vi "Drop Parameters.vi"(6 "Main UI Message Queue":refnum<queue>, 7 "Mouse Position":cluster{"X":i32, "Y":i32}, 8 "error in (no error)":errorcluster, 9 "Parent Window Title":string, 10 "Module Type":T1=enum."Feed", 11 "State in":T2 {"Main Config"."PR Module Configs"."Settings"."PID 2 Parameters"."output range"."output low" format="%.2f"; "Main Config"."PR Module Configs"."Settings"."PID 2 Parameters"."output range"."output high" min=0.0 max=100.0 format="%.2f"; "Main Config"."PR Module Configs"."Settings"."PID 2 Parameters"."PID gains"."derivative time (Td, min)" format="%.3f"; "Main Config"."PR Module Configs"."Settings"."PID 2 Parameters"."PID gains"."integral time (Ti, min)" format="%.3f"; "Main Config"."PR Module Configs"."Settings"."PID 2 Parameters"."PID gains"."proportional gain (Kc)" format="%.3f"; "Main Config"."Steps"."Control" items=["Pump %", "Setpoint"]; "Main Config"."TCU Module Configs"."Settings"."Huber Unistat 410 Settings"."Address" min=0 max=99 format="%02.0f"; "Main Config"."TCU Module Configs"."Settings"."Julabo FP-50 Settings"."Pump Power" min=0 max=8 step=1; "Main Config"."TCU Module Configs"."Settings"."Lauda Settings"."Pump Power" min=0 max=8 step=1; "Main Config"."Pump Module Configs"."Settings"."ASIA Pump C"."channel" min=0 max=1 step=1; "Main Config"."Pump Module Configs"."Settings"."Masterflex"."Pump Number" min=1.0 max=20.0 step=1.0; "Main Config"."Pump Module Configs"."Settings"."Ismatech"."Pump Number" min=1.0 max=20.0 step=1.0; "Main Config"."Feed Module Configs"."Settings"."output range"."output low" min=0.0 max=100.0 format="%.2f"; "Main Config"."Feed Module Configs"."Settings"."output range"."output high" format="%.2f"; "Main Config"."Feed Module Configs"."Settings"."PID 2 Parameters"."PID gains"."derivative time (Td, min)" format="%.3f"; "Main Config"."Feed Module Configs"."Settings"."PID 2 Parameters"."PID gains"."integral time (Ti, min)" format="%.3f"; "Main Config"."Feed Module Configs"."Settings"."PID 2 Parameters"."PID gains"."proportional gain (Kc)" format="%.3f"; "Main Config"."Feed Module Configs"."Settings"."ASIA Pump C"."channel" min=0 max=1 step=1; "Main Config"."Feed Module Configs"."Settings"."Ismatech"."Pump Number" min=1.0 max=20.0 step=1.0; "Main Config"."Feed Module Configs"."Settings"."Masterflex"."Pump Number" min=1.0 max=20.0 step=1.0}) -> (0 "error out":errorcluster, 2 "Drop Parameters":T66, 3 "State out":T2 {"Main Config"."PR Module Configs"."Settings"."PID 2 Parameters"."output range"."output low" format="%.2f"; "Main Config"."PR Module Configs"."Settings"."PID 2 Parameters"."output range"."output high" min=0.0 max=100.0 format="%.2f"; "Main Config"."PR Module Configs"."Settings"."PID 2 Parameters"."PID gains"."derivative time (Td, min)" format="%.3f"; "Main Config"."PR Module Configs"."Settings"."PID 2 Parameters"."PID gains"."integral time (Ti, min)" format="%.3f"; "Main Config"."PR Module Configs"."Settings"."PID 2 Parameters"."PID gains"."proportional gain (Kc)" format="%.3f"; "Main Config"."Steps"."Control" items=["Pump %", "Setpoint"]; "Main Config"."TCU Module Configs"."Settings"."Huber Unistat 410 Settings"."Address" min=0 max=99 format="%02.0f"; "Main Config"."TCU Module Configs"."Settings"."Julabo FP-50 Settings"."Pump Power" min=0 max=8 step=1; "Main Config"."TCU Module Configs"."Settings"."Lauda Settings"."Pump Power" min=0 max=8 step=1; "Main Config"."Pump Module Configs"."Settings"."ASIA Pump C"."channel" min=0 max=1 step=1; "Main Config"."Pump Module Configs"."Settings"."Masterflex"."Pump Number" min=1.0 max=20.0 step=1.0; "Main Config"."Pump Module Configs"."Settings"."Ismatech"."Pump Number" min=1.0 max=20.0 step=1.0; "Main Config"."Feed Module Configs"."Settings"."output range"."output low" min=0.0 max=100.0 format="%.2f"; "Main Config"."Feed Module Configs"."Settings"."output range"."output high" format="%.2f"; "Main Config"."Feed Module Configs"."Settings"."PID 2 Parameters"."PID gains"."derivative time (Td, min)" format="%.3f"; "Main Config"."Feed Module Configs"."Settings"."PID 2 Parameters"."PID gains"."integral time (Ti, min)" format="%.3f"; "Main Config"."Feed Module Configs"."Settings"."PID 2 Parameters"."PID gains"."proportional gain (Kc)" format="%.3f"; "Main Config"."Feed Module Configs"."Settings"."ASIA Pump C"."channel" min=0 max=1 step=1; "Main Config"."Feed Module Configs"."Settings"."Ismatech"."Pump Number" min=1.0 max=20.0 step=1.0; "Main Config"."Feed Module Configs"."Settings"."Masterflex"."Pump Number" min=1.0 max=20.0 step=1.0})   [LabVIEW 2018, in "Drag and Drop.lvlib"]
uses:
  Drag and Drop.lvlib
  Drop Parameters Cluster.ctl
  support/Message Queue/Message Cluster.ctl
  <vilib>/Utility/miscctls.llb/LVPoint32TypeDef.ctl
  State Cluster.ctl
  Thumbnail Cluster.ctl
  Object Cluster.ctl
  <vilib>/Utility/miscctls.llb/LVRectTypeDef.ctl
  Object Type Enum.ctl
  <vilib>/Utility/miscctls.llb/LVPositionTypeDef.ctl
  Config Module/Controls/Main Config Cluster.ctl
  OPC/OPC Module Config.ctl
  Scale Module Folder/Measure Instrument/State Enum.ctl
  OPC/OPC Settings.ctl
  OPC/Variable Data Cluster.ctl
  <vilib>/OPCUA/controls/NodeId.ctl
  <vilib>/OPCUA/controls/OPC UA StatusCode.ctl
  <vilib>/OPCUA/controls/Subscription ID.ctl
  <vilib>/OPCUA/controls/OPC UA Client Refnum.ctl
  <vilib>/OPCUA/controls/Subscription Data Change.ctl
  <vilib>/OPCUA/controls/Data Type.ctl
  Feed Module/Controls/Feed Module Config Cluster.ctl
  Feed Module/Controls/Feed Module Settings Cluster.ctl
  Ismatec ISM 831C/Controls/Ismatech Settings Cluster.ctl
  Masterflex 7550-30/Controls/Settings Cluster.ctl
  Mettler Toledo/Controls/Settings Cluster.ctl
  Bronkhorst M13 Flow Meter/Settings Cluster.ctl
  Measure Instrument/PID 2 Parameters Cluster.ctl
  Measure Instrument/PID Input Enum.ctl
  Measure Instrument/PID 2 Output Enum.ctl
  Tacmina QI/Tacmina QI DAQ Setting.ctl
  KNF Pump/Settings Cluster plus SIMDOS.ctl
  ASIA Pump/Pump Settings.ctl
  VICI M50 Party Mode/Settings Cluster.ctl
  FLOM Pump/Settings Cluster.ctl
  SSI PR Class/SSI PR or LD Settings Cluster.ctl
  Masterflex 75211/Masterflex 75211 DAQ Setting.ctl
  SSI PR Class/SSI P40 Settings Cluster.ctl
  TT Module/Controls/TT Module Config Cluster.ctl
  Tag VIs/Numeric Alarm Settings Cluster.ctl
  Acquisition/Hardware Configuration.ctl
  Acquisition/Task Cluster.ctl
  PT Module/Controls/PT Module Config Cluster.ctl
  Scale Module Folder/Feed Module/Controls/Scale Module Config Cluster.ctl
  Scale Module Folder/Feed Module/Controls/Scale Module Settings Cluster.ctl
  Pump Module Folder/Pump Module Config Cluster.ctl
  Pump Module Folder/Pump Module Settings Cluster.ctl
  LabJack Module/Controls/U3 Module Config Cluster.ctl
  Decoration Module/Decoration Module Config Cluster.ctl
  Flow Module Folder/Feed Module/Controls/Flow Module Config Cluster.ctl
  Flow Module Folder/Feed Module/Controls/Flow Module Settings Cluster.ctl
  TCU Module/TCU Module Folder/TCU Module Config Cluster.ctl
  TCU Module/TCU Module Folder/TCU Module Settings Cluster.ctl
  TCU Module/TCU Module Folder/Measure Instrument/Output Devices.ctl
  Huber TCU/Huber Settings.ctl
  Lauda Integral XT-150 TCU/Lauda Settings.ctl
  Julabo Type 1 TCU/Julabo Type 1 TCU Folder/Julabo FP-50 Settings.ctl
  Huber Unistat 410 TCU/Huber Unistat 410 RS485 Settings.ctl
  D-O Module Folder/Not Sure Where this is Used.ctl
  Sequencing/Squence Control.ctl
  D-O Module Folder/D-O Module Config Cluster.ctl
  D-O Module Folder/Valve Clusters.ctl
  D-O Module Folder/D-O Module Settings Cluster.ctl
  D-O Module Folder/D-O Device Settings Cluster.ctl
  VICI Electronic Actuator/VICI Electronic Actuator Settings.ctl
  Pressure Regulator Control Module/Pressure Regulator/Controls/4-20mA Module Config Cluster.ctl
  Pressure Regulator Control Module/Pressure Regulator/Controls/4-20mA Module Settings Cluster.ctl
  Pressure Transmitter/Pressure Transmitter Device Settings.ctl
  Pressure Reg Module/Pressure Regulator Device Settings.ctl
  Module Type Enum.ctl
  Module Instance Number Operation Enum.ctl
  Flow Module Folder/Flow Module (Main).vi
  D-O Module Folder/D-O Module (Main).vi
  TCU Module/TCU Module Folder/TCU Module (Main).vi
  LabJack Module/U3 (Main).vit
  Feed Module/Feed Module.lvlib
  TT Module/TT Module.lvlib
  support/Message Queue/Message Queue.lvlib
  Bronkhorst M13 Flow Meter/Bronkhorst M13 Flow Meter.lvlib
  Mettler Toledo/Mettler Toledo.lvlib
  Masterflex 7550-30/Masterflex 7550-30.lvlib
  Ismatec ISM 831C/Ismatec ISM 831C.lvlib
  PT Module/PT Module.lvlib
  Shared Variables/Dynamic Shared Variables.lvlib
  Scale Module Folder/Scale Module.lvlib
  Pump Module Folder/Pump Module.lvlib
  LabJack Module/U3 Module.lvlib
  Flow Module Folder/Flow Module.lvlib
  Tacmina QI/Tacmina QI.lvlib
  KNF Pump/KNF SIMDOS.lvlib
  TCU Module/TCU Module Folder/TCU Module.lvlib
  Huber TCU/Huber Ministat 230 TCU.lvlib
  Lauda Integral XT-150 TCU/Lauda TCU.lvlib
  Julabo Type 1 TCU/Julabo Type 1 TCU Folder/Julabo Type FP-50 TCU.lvlib
  ASIA Pump.lvlib
  VICI M50 Party Mode/VICI M6 M50 Party Mode.lvlib
  D-O Module Folder/D-O Module.lvlib
  Pressure Regulator Control Module/Pressure Regulator/4-20mA Module.lvlib
  Pressure Transmitter/Pressure Transmitter Library.lvlib
  Pressure Reg Module/Pressure Regulator Library.lvlib
  FLOM Pump/FLOM Pump.lvlib
  SSI PR Class/SSI PR or LD Pump.lvlib
  OPC/OPC UA.lvlib
  Scale Module Folder/Measure Instrument/Scale Module Engine.lvlib
  D-O Module Folder/DIO Valve/VICI Electronic Actuator.lvlib
  Masterflex 75211/Masterflex 75211.lvlib
  SSI PR Class/SSI P40 Pump.lvlib
  Huber Unistat 410 TCU/Huber Unistat 410 TCU.lvlib
  Config Module/Config Module.lvlib
  DAQ/DAQ.lvlib
  Sequencing/Sequencing Library.lvlib
panel:
  # "Instrument Settings"
  # "Instrument Settings"
  # "Output Instruments"
  # "Flow Meter Settings"
  # "Output Instruments"
  # "Scale Settings"
  # "Output Instruments"
  # "Input Instruments"
  # "Instrument Settings"
  # "Instrument Settings"
  # "Output Instruments"
  # "Flow Meter Settings"
  # "Output Instruments"
  # "Scale Settings"
  # "Output Instruments"
  # "Input Instruments"
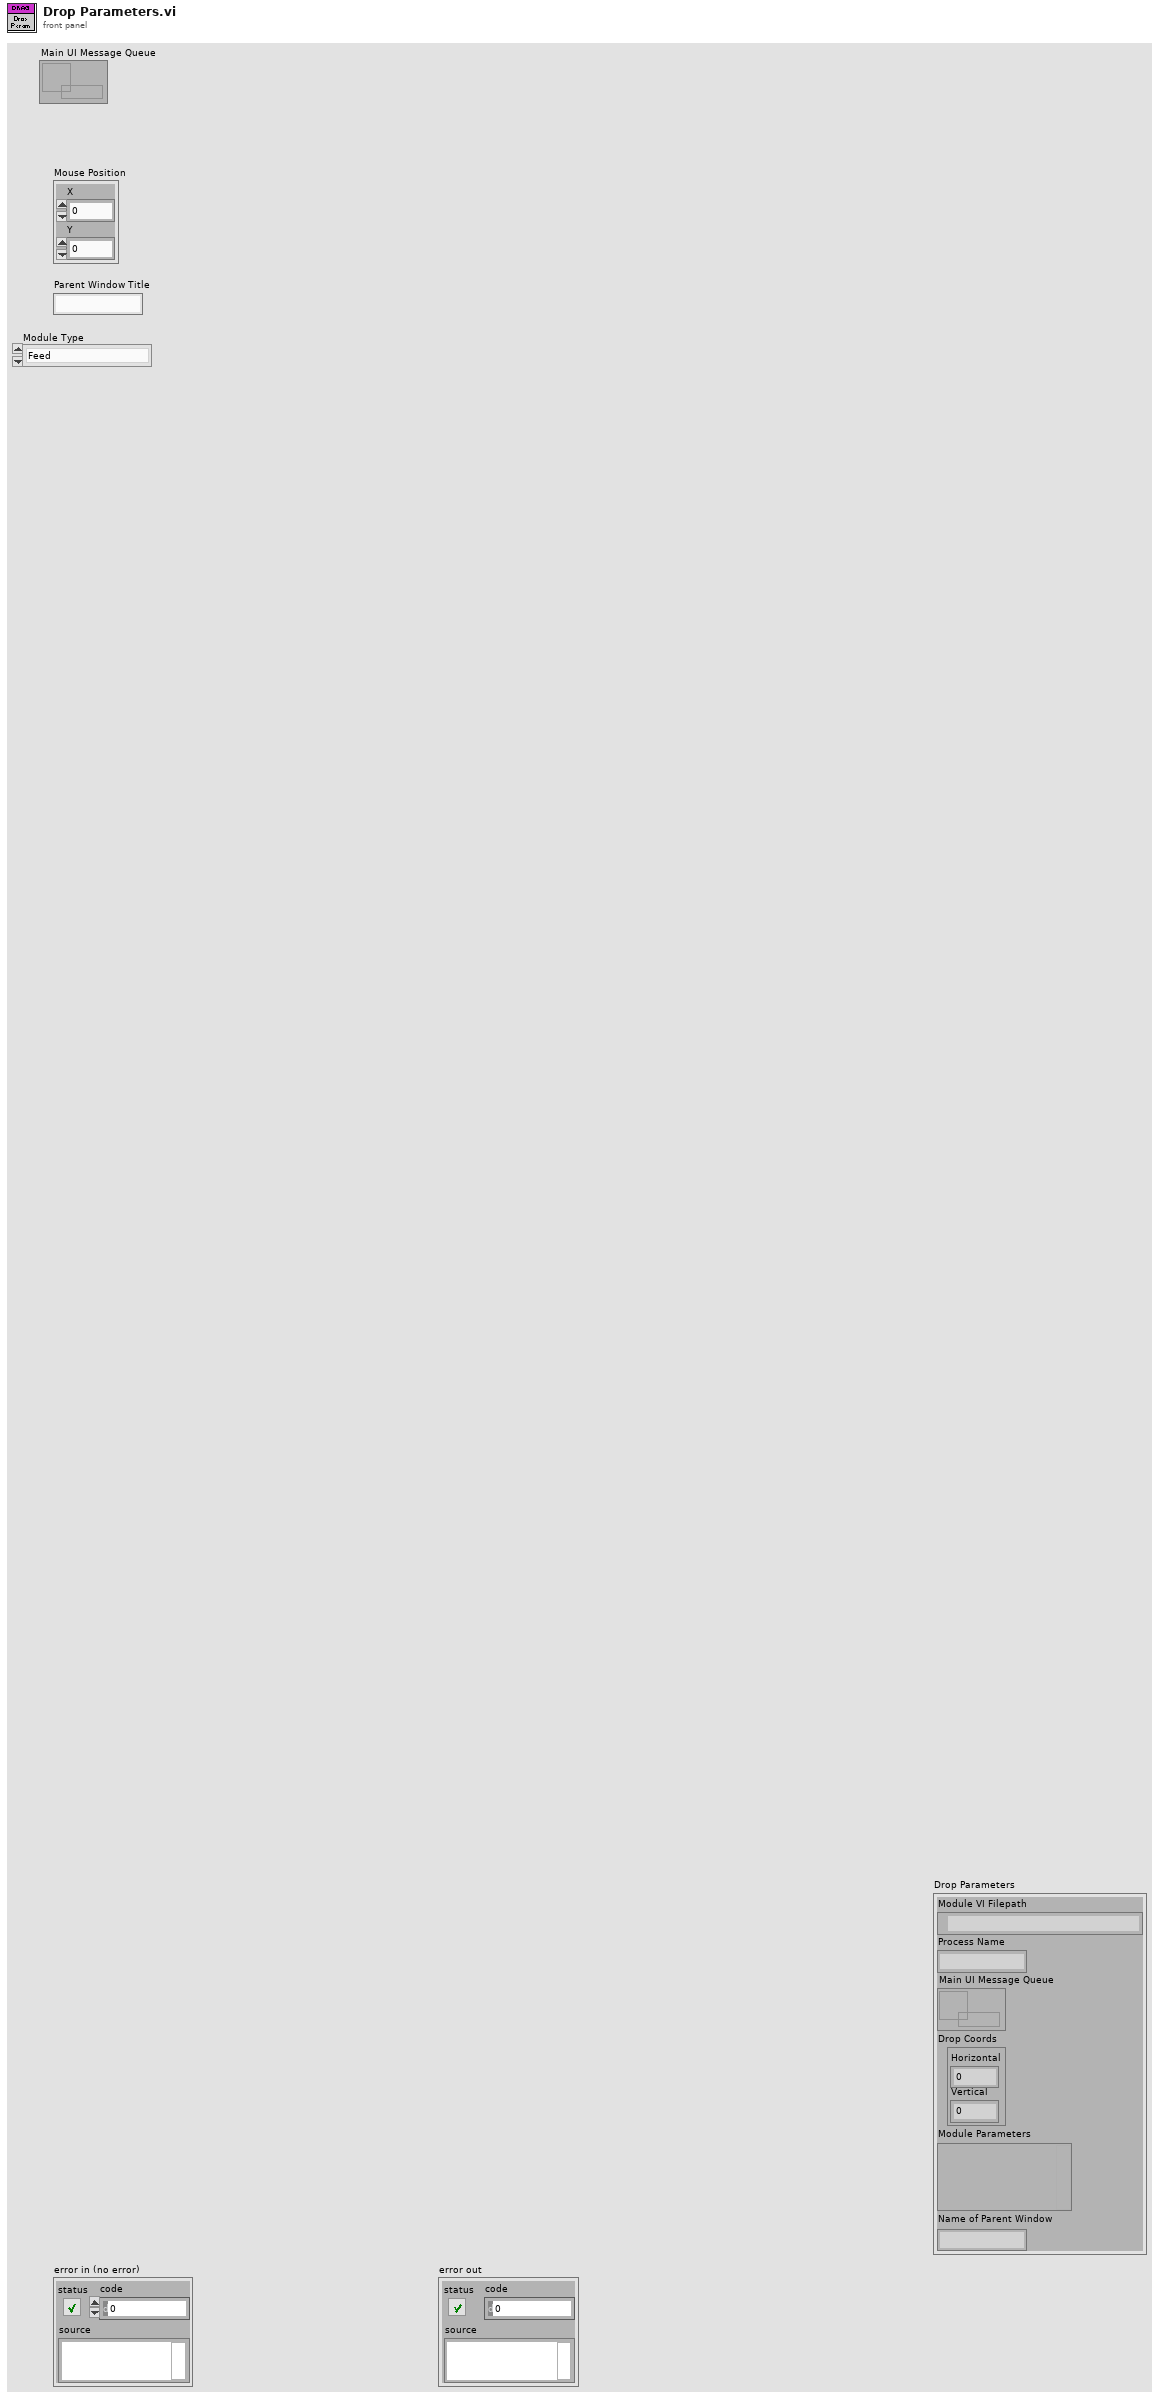
[diagram p1: front panel]
types:
  T1 = typedef "Drag and Drop.lvlib/Module Type Enum.ctl" = enum16{"<unknown module>", "Feed", "TT", "PT", "Scale", "Flow", "Pump", "U3", "TCU", "DO", "PR", "OPC"}
  T2 = typedef "Drag and Drop.lvlib/State Cluster.ctl" = cluster{"VI refs":refnum<vi>[], "Queues":refnum<queue>[], "[Thumbnails]":T3[], "Drag Object Idx":i32, "[Objects]":T4[], "Active Object":i32, "Drop Offset":T7, "Process Name":string, "Main Config":T8, "Campaign Filepath":path, "Config Changed?":bool}
  T3 = typedef "Thumbnail Cluster.ctl" = cluster{"Path":path, "Rectangle":cluster{"left":i16, "top":i16, "right":i16, "bottom":i16}}
  T4 = typedef "Object Cluster.ctl" = cluster{"BMP Path":path, "Anchor Position":cluster{"X":i32, "Y":i32}, "Hot Spot":T5, "Type":T6, "Parameters":variant}
  T5 = typedef "LVRectTypeDef.ctl" = cluster{"Left":i16, "Top":i16, "Right":i16, "Bottom":i16}
  T6 = typedef "Object Type Enum.ctl" = enum16{"Icon", "Line", "Text", "Feed Module"}
  T7 = typedef "LVPositionTypeDef.ctl" = cluster{"Left":i32, "Top":i32}
  T8 = typedef "Config Module.lvlib/Main Config Cluster.ctl" = cluster{"Notebook":string, "Page":string, "OPC Module Configs":T9[], "Feed Module Configs":T18[], "Log File Path":path, "TT Module Configs":T35[], "DAQ Config":T37, "PT Module Configs":T39[], "Scale Module Configs":T40[], "Pump Module Configs":T42[], "U3 Module Configs":T44[], "Decoration Module Configs":T45[], "Flow Module Configs":T46[], "TCU Module Configs":T48[], "Steps":T55, "Abort":bool, "DO Module Configs":T57[], "PR Module Configs":T62[], "Cycle Period":dbl}
  T9 = typedef "OPC UA.lvlib/OPC Module Config.ctl" = cluster{"State":T10, "GUID":string, "Drop Coords":T11, "Configuration":T12, "First Iteration":bool, "Data":cluster{"Object Name":string, "Variable Array":T13[]}[], "Process Name":string, "Load Count":i32, "Log Started":bool, "subscription ID out":T16, "OPC UA client refnum out":T17, "Event Registration Refnum":refnum<event-registration>, "Start Time":timestamp, "Current Time":timestamp}
  T10 = typedef "Scale Module.lvlib/Scale Module Engine.lvlib/State Enum.ctl" = enum16{"Measuring", "Idle"}
  T11 = typedef "LVPoint32TypeDef.ctl" = cluster{"Horizontal":i32, "Vertical":i32}
  T12 = typedef "OPC UA.lvlib/OPC Settings.ctl" = cluster{"Cycle Period":dbl, "server endpoint URL":string, "security policy":cluster{"message mode":enum16{"None", "Sign", "Sign and Encrypt"}, "security":enum16{"Basic256", "Basic128Rsa15"}}, "Trust Any Server":bool}
  T13 = typedef "OPC UA.lvlib/Variable Data Cluster.ctl" = cluster{"node ID":T14, "browse name":string, "status":T15, "timestamp":timestamp, "value ":variant}
  T14 = typedef "NodeId.ctl" = string
  T15 = typedef "OPC UA StatusCode.ctl" = u32
  T16 = typedef "Subscription ID.ctl" = u32
  T17 = typedef "OPC UA Client Refnum.ctl" = refnum<k21>
  T18 = typedef "Feed Module.lvlib/Feed Module Config Cluster.ctl" = cluster{"GUID":string, "Drop Coords":T11, "Process Name":string, "Queue Name":string, "Settings":T19, "Settings Load Count":i32, "OP Load Count":i32}
  T19 = typedef "Feed Module.lvlib/Feed Module Settings Cluster.ctl" = cluster{"Cycle Period":dbl, "Ismatech":T20, "Masterflex":T21, "Mettler":T22, "Bronkhorst M13 Flow Meter":T23, "PID 2 Parameters":T24, "Manual Entry":dbl, "Auto?":bool, "output range":cluster{"output high":dbl, "output low":dbl}, "Bronkhorst M14":T22, "Tacmina Settings":T27, "KNF SIMDOS Settings":T28, "ASIA Pump C":T29, "VICI Settings":T30, "FLOM Settings":T31, "SSI PR/LD Settings":T32, "Masterflex 75211 Settings":T33, "SSI P40 Settings":T34}
  T20 = typedef "Ismatec ISM 831C.lvlib/Ismatech Settings Cluster.ctl" = cluster{"VISA resource name":refnum<visa-resource-name>, "Simulated?":bool, "Pump Number":dbl, "Reverse?":bool}
  T21 = typedef "Masterflex 7550-30.lvlib/Settings Cluster.ctl" = cluster{"VISA resource name":refnum<visa-resource-name>, "Simulated?":bool, "Pump Number":dbl, "Reverse?":bool}
  T22 = typedef "Mettler Toledo.lvlib/Settings Cluster.ctl" = cluster{"VISA resource name":refnum<visa-resource-name>, "Simulated?":bool}
  T23 = typedef "Bronkhorst M13 Flow Meter.lvlib/Settings Cluster.ctl" = cluster{"VISA resource name":refnum<visa-resource-name>, "Simulated?":bool}
  T24 = typedef "PID 2 Parameters Cluster.ctl" = cluster{"Input Device":T25, "Output Device":T26, "Setpoint":dbl, "PID gains":cluster{"proportional gain (Kc)":dbl, "integral time (Ti, min)":dbl, "derivative time (Td, min)":dbl}}
  T25 = typedef "PID Input Enum.ctl" = enum16{"Default", "Bronkhorst M13", "Bronkhorst M14", "Scale Rate of Change"}
  T26 = typedef "PID 2 Output Enum.ctl" = enum16{"Default", "Ismatec ISM 831C", "Masterflex 7550-30", "VICI", "Tacmina QI", "KNF SIMDOS", "ASIA Type C", "FLOM UI-22-11", "SSI PR/LD", "SSI P40", "Masterflex 75211-70"}
  T27 = typedef "Tacmina QI.lvlib/Tacmina QI DAQ Setting.ctl" = cluster{"Analog DAQ Task":refnum<k21>, "Digital DAQ Task":refnum<k21>}
  T28 = typedef "KNF SIMDOS.lvlib/Settings Cluster plus SIMDOS.ctl" = cluster{"VISA resource name":refnum<visa-resource-name>, "Simulated?":bool}
  T29 = typedef "ASIA Pump.lvlib/Pump Settings.ctl" = cluster{"ASIA Pump #":i32, "channel":i32, "Simulated":bool}
  T30 = typedef "VICI M6 M50 Party Mode.lvlib/Settings Cluster.ctl" = cluster{"VISA resource name":refnum<visa-resource-name>, "Simulated?":bool, "Pump Letter":string, "Reverse?":bool}
  T31 = typedef "FLOM Pump.lvlib/Settings Cluster.ctl" = cluster{"VISA resource name":refnum<visa-resource-name>, "Simulated?":bool, "Pump Number":dbl}
  T32 = typedef "SSI PR or LD Pump.lvlib/SSI PR or LD Settings Cluster.ctl" = cluster{"VISA resource name":refnum<visa-resource-name>, "Simulated?":bool}
  T33 = typedef "Masterflex 75211.lvlib/Masterflex 75211 DAQ Setting.ctl" = cluster{"Analog DAQ Task":refnum<k21>, "Digital DAQ Task":refnum<k21>}
  T34 = typedef "SSI P40 Pump.lvlib/SSI P40 Settings Cluster.ctl" = cluster{"VISA resource name":refnum<visa-resource-name>, "Simulated?":bool}
  T35 = typedef "TT Module.lvlib/TT Module Config Cluster.ctl" = cluster{"GUID":string, "Drop Coords":T11, "Input Channel Tag Name ":string, "Process Name":string, "Queue Name":string, "Input Channel Numeric Alarm Settings":T36[]}
  T36 = typedef "Numeric Alarm Settings Cluster.ctl" = cluster{"enable? (F)":bool, "name":string, "alarm type":enum16{"HI_HI", "HI", "LO", "LO_LO"}, "level/change":dbl, "deadband/time":dbl, "alarm delay":dbl, "priority":u32, "ack type":enum16{"Auto", "User", "None", "Each Occurrence"}, "area":string, "description":string, "log? (T)":bool}
  T37 = typedef "DAQ.lvlib/Hardware Configuration.ctl" = cluster{"Tasks":T38[]}
  T38 = typedef "Task Cluster.ctl" = cluster{"DAQmx Task":refnum<k21>, "Read-Write Radio":enum32{"Read", "Write"}}
  T39 = typedef "PT Module.lvlib/PT Module Config Cluster.ctl" = cluster{"GUID":string, "Drop Coords":T11, "Input Channel Tag Name ":string, "Process Name":string, "Queue Name":string, "Input Channel Numeric Alarm Settings":T36[]}
  T40 = typedef "Scale Module.lvlib/Scale Module Config Cluster.ctl" = cluster{"GUID":string, "Drop Coords":T11, "Process Name":string, "Queue Name":string, "Settings":T41, "Load Count":i32}
  T41 = typedef "Scale Module.lvlib/Scale Module Settings Cluster.ctl" = cluster{"Cycle Period":dbl, "Mettler":T22, "Scale Type":string}
  T42 = typedef "Pump Module.lvlib/Pump Module Config Cluster.ctl" = cluster{"GUID":string, "Drop Coords":T11, "Process Name":string, "Queue Name":string, "Settings":T43, "Load Count":i32}
  T43 = typedef "Pump Module.lvlib/Pump Module Settings Cluster.ctl" = cluster{"Cycle Period":dbl, "Manual Entry":dbl, "Output Device":T26, "Ismatech":T20, "Masterflex":T21, "VICI Settings":T30, "Tacmina Settings":T27, "KNF SIMDOS Settings":T28, "ASIA Pump C":T29, "FLOM Settings":T31, "SSI PR/LD Settings":T32, "SSI P40 Settings":T32, "Masterflex 75211 Settings":T33, "Pump Calibration File":path, "Calibration Slope":dbl, "Calibration Y Intercept":dbl, "Pump Cal Enum":u16}
  T44 = typedef "U3 Module.lvlib/U3 Module Config Cluster.ctl" = cluster{"GUID":string, "Drop Coords":T11, "AI Channel Number":enum16{"Default", "AI0", "AI1", "AI2", "AI3", "AI4", "AI5", "AI6", "AI7"}, "Process Name":string, "Queue Name":string, "Input Channel Numeric Alarm Settings":T36[]}
  T45 = typedef "Decoration Module Config Cluster.ctl" = cluster{"GUID":string, "Drop Coords":T11, "Decoration Filepath":path}
  T46 = typedef "Flow Module.lvlib/Flow Module Config Cluster.ctl" = cluster{"GUID":string, "Drop Coords":T11, "Process Name":string, "Queue Name":string, "Settings":T47, "Load Count":i32}
  T47 = typedef "Flow Module.lvlib/Flow Module Settings Cluster.ctl" = cluster{"Cycle Period":dbl, "Bronkhorst M13":T22, "Flow Meter Type":string, "Bronkhorst M14":T22}
  T48 = typedef "TCU Module.lvlib/TCU Module Config Cluster.ctl" = cluster{"GUID":string, "Drop Coords":T11, "Process Name":string, "Queue Name":string, "Settings":T49, "Load Count":i32, "Power Level Changed":bool}
  T49 = typedef "TCU Module.lvlib/TCU Module Settings Cluster.ctl" = cluster{"Cycle Period":dbl, "Setpoint Entry":dbl, "Output Device":T50, "Huber Ministat 230 Settings":T51, "Lauda Settings":T52, "Julabo FP-50 Settings":T53, "Internal Control?":bool, "Huber Unistat 410 Settings":T54}
  T50 = typedef "Output Devices.ctl" = enum16{"Default", "Huber Ministat 230", "Huber Unistat 410", "Lauda XT-150", "Julabo FP-50"}
  T51 = typedef "Huber Ministat 230 TCU.lvlib/Huber Settings.ctl" = cluster{"VISA resource name":refnum<visa-resource-name>, "Simulated?":bool}
  T52 = typedef "Lauda TCU.lvlib/Lauda Settings.ctl" = cluster{"VISA resource name":refnum<visa-resource-name>, "Simulated?":bool, "Pump Power":i32}
  T53 = typedef "Julabo Type FP-50 TCU.lvlib/Julabo FP-50 Settings.ctl" = cluster{"VISA resource name":refnum<visa-resource-name>, "Simulated?":bool, "Pump Power":i32}
  T54 = typedef "Huber Unistat 410 TCU.lvlib/Huber Unistat 410 RS485 Settings.ctl" = cluster{"VISA resource name":refnum<visa-resource-name>, "Address":i8, "Simulated?":bool}
  T55 = typedef "Not Sure Where this is Used.ctl" = T56[]
  T56 = typedef "Sequencing Library.lvlib/Squence Control.ctl" = cluster{"Module":string, "Control":u16, "Value":dbl, "Wait (sec)":dbl}
  T57 = typedef "D-O Module.lvlib/D-O Module Config Cluster.ctl" = cluster{"GUID":string, "Drop Coords":T11, "Process Name":string, "Queue Name":string, "Settings":T58, "Load Count":i32}
  T58 = typedef "D-O Module.lvlib/Valve Clusters.ctl" = cluster{"Valve Settings":T59, "Valve Type":enum16{"Default", "Digital Output Valve", "VICI Electronic Actuator"}, "Time On (Sec)":dbl, "Time Off (Sec)":dbl, "Run?":bool}
  T59 = typedef "D-O Module.lvlib/D-O Module Settings Cluster.ctl" = cluster{"D-O Settings":T60, "VICI Electronic Actuator":T61}
  T60 = typedef "D-O Module.lvlib/D-O Device Settings Cluster.ctl" = cluster{"DAQmx Task Name":refnum<k21>, "Output Channel":u16, "Output Channel Names":string[]}
  T61 = typedef "VICI Electronic Actuator.lvlib/VICI Electronic Actuator Settings.ctl" = cluster{"VISA resource name":refnum<visa-resource-name>, "Mode":enum16{"Two Positions With Stops", "Two Positions Without Stops", "Mutiposition"}, "Simulated":bool}
  T62 = typedef "4-20mA Module.lvlib/4-20mA Module Config Cluster.ctl" = cluster{"GUID":string, "Drop Coords":T11, "Process Name":string, "Queue Name":string, "Settings":T63, "Settings Load Count":i32}
  T63 = typedef "4-20mA Module.lvlib/4-20mA Module Settings Cluster.ctl" = cluster{"Cycle Period":dbl, "PID 2 Parameters":cluster{"Input Device":enum16{"Default", "4-20mA"}, "Output Device":enum16{"Default", "Equilibar Pressure Reg", "Flow Regulator"}, "Setpoint":dbl, "PID gains":cluster{"proportional gain (Kc)":dbl, "integral time (Ti, min)":dbl, "derivative time (Td, min)":dbl}, "output range":cluster{"output low":dbl, "output high":dbl}}, "Manual Entry":dbl, "Auto?":bool, "4-20mA Input Settings":T64, "4-20mA Out Settings":T65, "Input Channel Tag Name ":string}
  T64 = typedef "Pressure Transmitter Library.lvlib/Pressure Transmitter Device Settings.ctl" = cluster{"Input Channel ":u16}
  T65 = typedef "Pressure Regulator Library.lvlib/Pressure Regulator Device Settings.ctl" = cluster{"Output DAQ Task":refnum<k21>}
  T66 = typedef "Drop Parameters Cluster.ctl" = cluster{"Module VI Filepath":path, "Process Name":string, "Main UI Message Queue":refnum<queue>, "Drop Coords":T11, "Module Parameters":variant, "Name of Parent Window":string}
  T67 = typedef "Module Instance Number Operation Enum.ctl" = enum16{"Init", "Next Instance Number"}
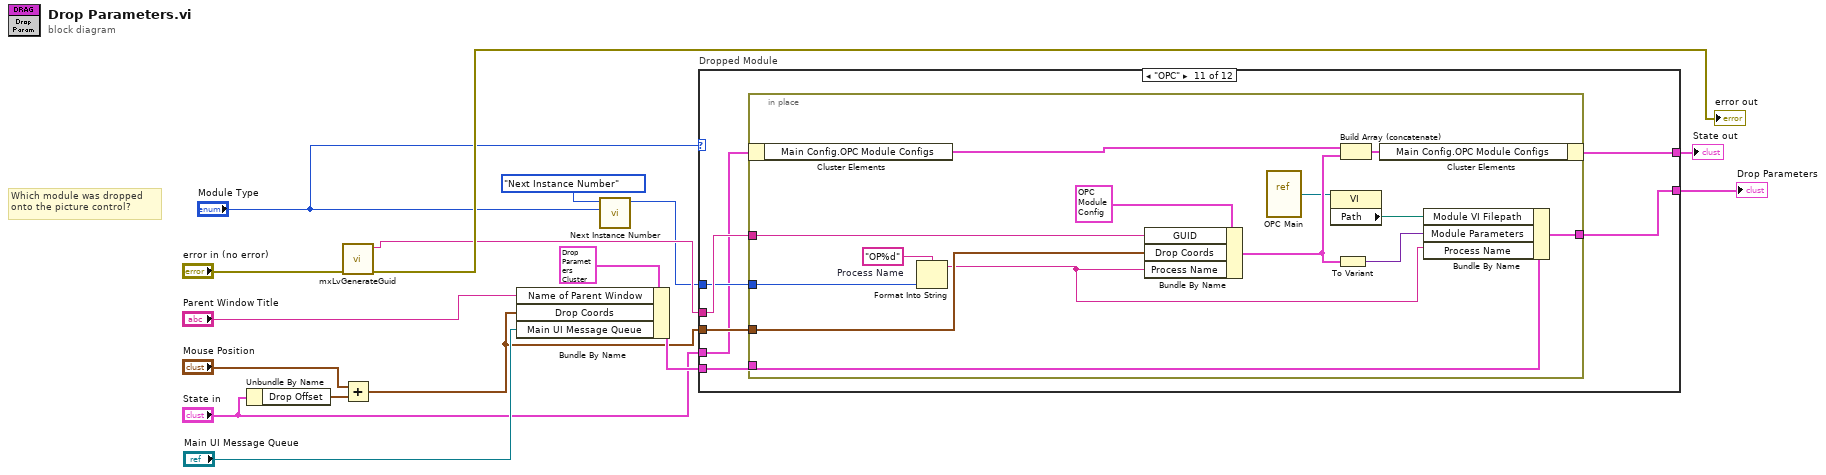
[diagram p0: block diagram]
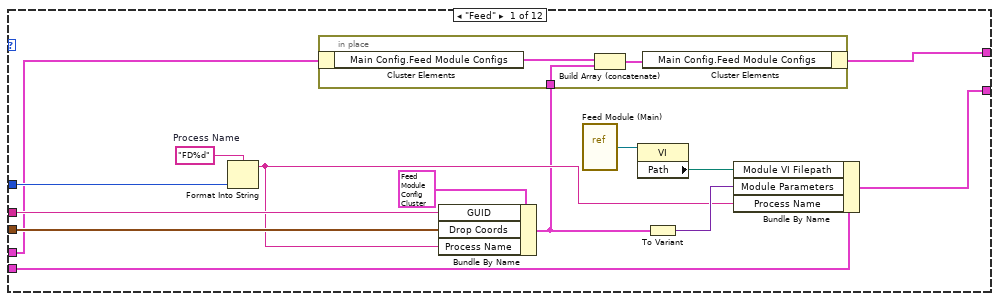
[diagram p2: hidden frame]
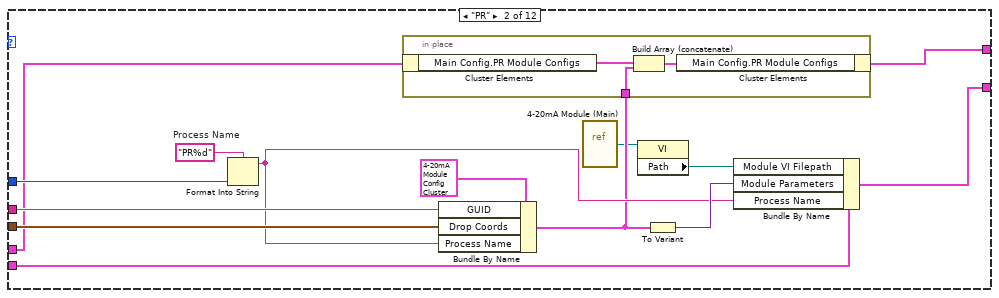
[diagram p3: hidden frame]
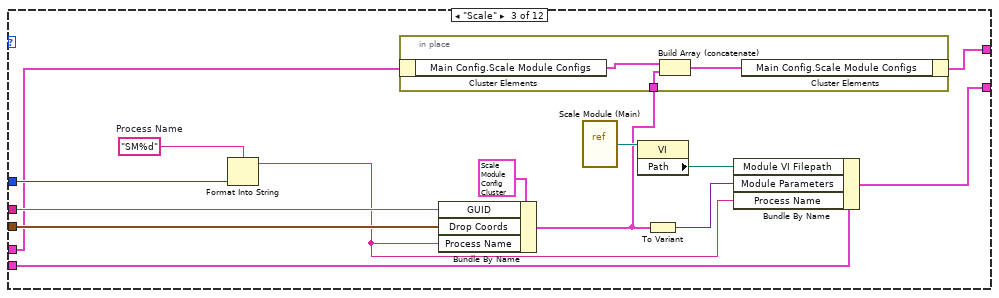
[diagram p4: hidden frame]
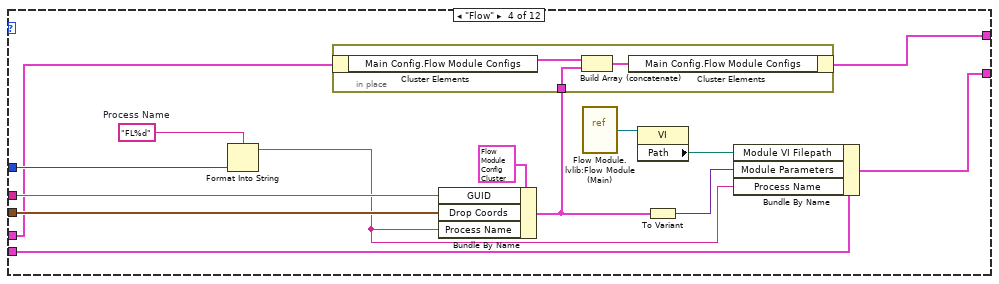
[diagram p5: hidden frame]
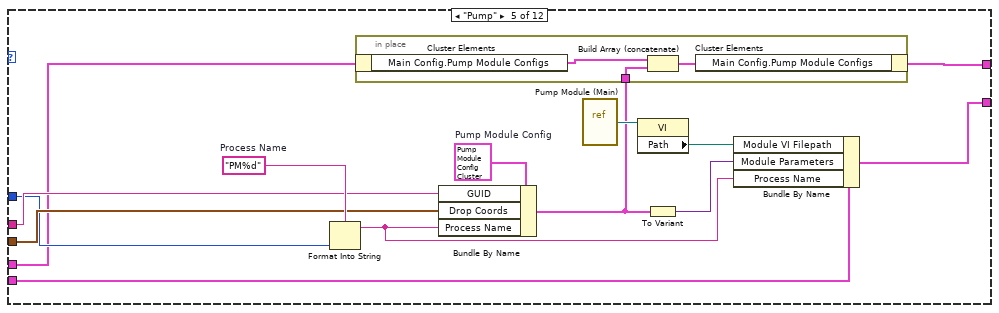
[diagram p6: hidden frame]
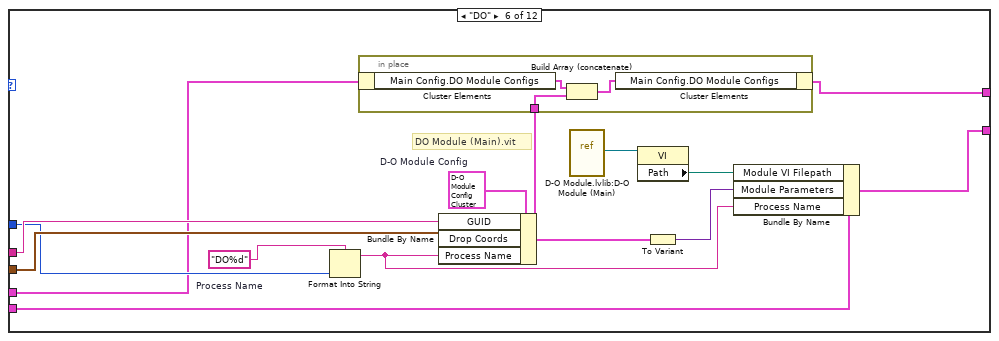
[diagram p7: hidden frame]
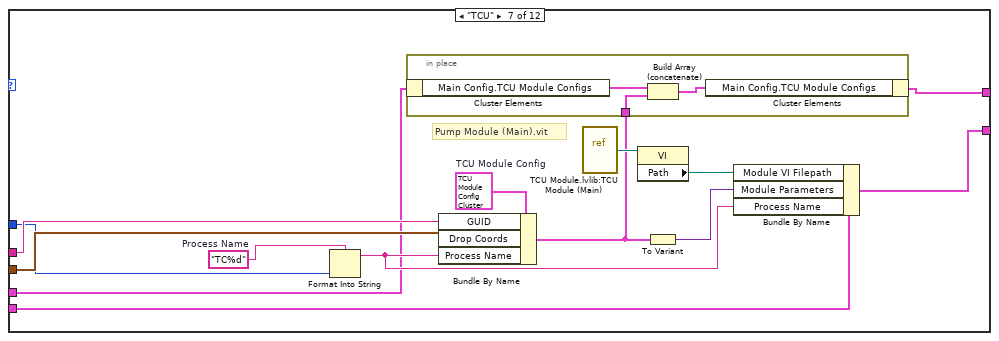
[diagram p8: hidden frame]
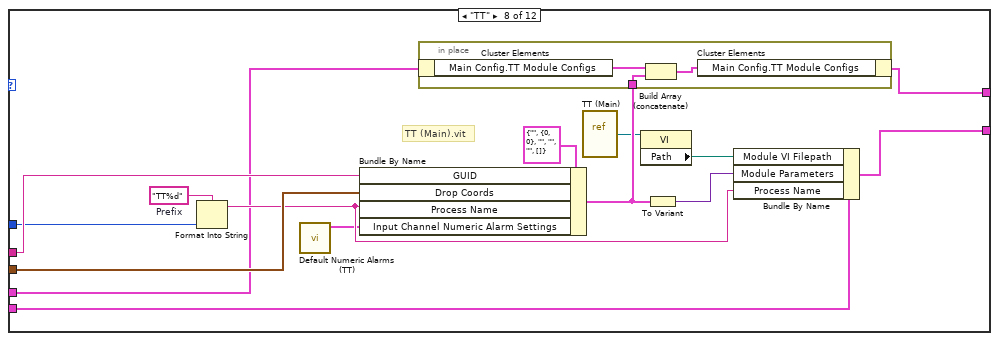
[diagram p9: hidden frame]
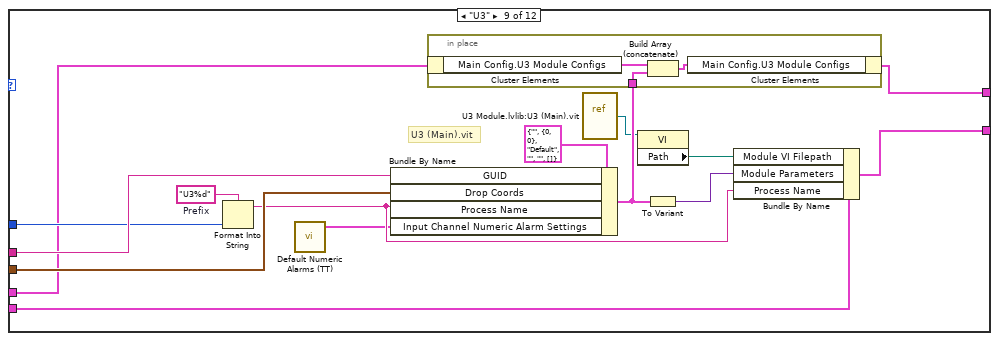
[diagram p10: hidden frame]
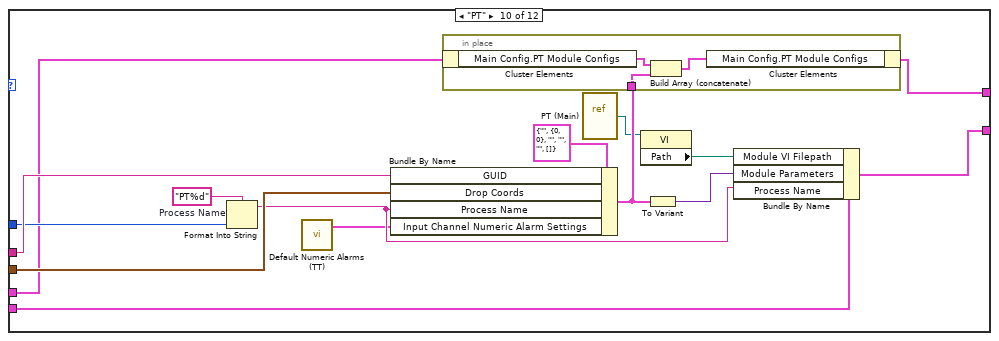
[diagram p11: hidden frame]
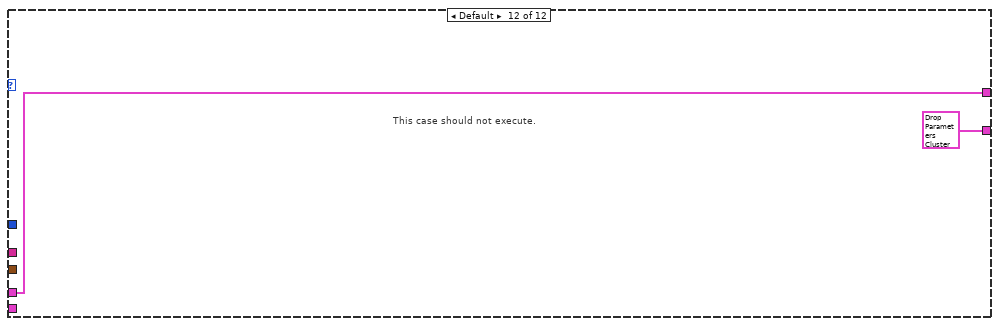
[diagram p12: hidden frame]
diagram:
  # "Which module was dropped\nonto the picture control?"
  n1 = Unbundle By Name("State in") -> ("Drop Offset"=w12:T7)
  n2 = call <resource>:"mxLvGenerateGuid.vi"("Error In"="error in (no error)") -> ("Error Out"=→"error out":errorcluster, "Value"=w13:string)  [unwired: 9 in]
  n3 = Add(x="Mouse Position", y=w12) -> (x+y=w6:T7)
  n4 = Bundle By Name(cluster=T66 {"Module VI Filepath"=path "", "Process Name"="", "Main UI Message Queue"=refnum, "Drop Coords"={"Horizontal"=0, "Vertical"=0}, "Module Parameters"=variant, "Name of Parent Window"=""} ("Drop Parameters"), "Name of Parent Window"="Parent Window Title", "Drop Coords"=w6, "Main UI Message Queue"="Main UI Message Queue") -> (w8:T66)
  n5 = call "Next Instance Number.vi"("Module Type"="Module Type", "Operation"=Module_Instance_Number_Operation_Enum."Next Instance Number") -> ("Instance Number"=w3:i32)  [unwired: 8 in, 1 out]
  n6 = case "Dropped Module" shown="\"OPC\"" "Module Type" {
    tunnel: "State in" -> [w18 w35 w52 w69 w86 w103 w120 w136 w155 w173 w191 w212]
    tunnel: [w17 w34 w51 w68 w85 w102 w119 w137 w154 w172 w190 w212] -> w2
    tunnel: [w28 w45 w62 w79 w97 w114 w131 w149 w167 w185 w192 T66 {"Module VI Filepath"=path "", "Process Name"="", "Main UI Message Queue"=refnum, "Drop Coords"={"Horizontal"=0, "Vertical"=0}, "Module Parameters"=variant, "Name of Parent Window"=""} ("Drop Parameters")] -> w16
    tunnel: w13 -> [w27 w44 w61 w78 w96 w113 w130 w148 w166 w184 w196 _]
    tunnel: w8 -> [w26 w43 w60 w77 w95 w112 w129 w147 w165 w183 w195 _]
    tunnel: w6 -> [w24 w41 w58 w75 w93 w110 w127 w145 w163 w181 w194 _]
    tunnel: w3 -> [w19 w36 w54 w71 w89 w106 w123 w139 w157 w175 w193 _]
    frame "Feed" {
      w29 = "FD%d"  # Process Name
      n7 = Format Into String(format string=w29, w19) -> (resulting string=w23:string)  [unwired: 2 in, 1 out]
      n8 = Bundle By Name(cluster=T18 {"GUID"="", "Drop Coords"={"Horizontal"=0, "Vertical"=0}, "Process Name"="", "Queue Name"="", "Settings"={"Cycle Period"=500.0, "Ismatech"={"VISA resource name"="", "Simulated?"=TRUE, "Pump Number"=1.0, "Reverse?"=FALSE}, "Masterflex"={"VISA resource name"="", "Simulated?"=TRUE, "Pump Number"=1.0, "Reverse?"=FALSE}, "Mettler"={"VISA resource name"="", "Simulated?"=FALSE}, "Bronkhorst M13 Flow Meter"={"VISA resource name"="", "Simulated?"=TRUE}, "PID 2 Parameters"={"Input Device"=enum."Default", "Output Device"=enum."Default", "Setpoint"=0.0, "PID gains"={"proportional gain (Kc)"=1.0, "integral time (Ti, min)"=0.01, "derivative time (Td, min)"=0.0}}, "Manual Entry"=0.0, "Auto?"=TRUE, "output range"={"output high"=100.0, "output low"=0.0}, "Bronkhorst M14"={"VISA resource name"="", "Simulated?"=FALSE}, "Tacmina Settings"={"Analog DAQ Task"="", "Digital DAQ Task"=""}, "KNF SIMDOS Settings"={"VISA resource name"="", "Simulated?"=TRUE}, "ASIA Pump C"={"ASIA Pump #"=0, "channel"=0, "Simulated"=FALSE}, "VICI Settings"={"VISA resource name"="", "Simulated?"=TRUE, "Pump Letter"="", "Reverse?"=FALSE}, "FLOM Settings"={"VISA resource name"="", "Simulated?"=TRUE, "Pump Number"=0.0}, "SSI PR/LD Settings"={"VISA resource name"="", "Simulated?"=FALSE}, "Masterflex 75211 Settings"={"Analog DAQ Task"="", "Digital DAQ Task"=""}, "SSI P40 Settings"={"VISA resource name"="", "Simulated?"=TRUE}}, "Settings Load Count"=0, "OP Load Count"=0} ("Feed Module Config"), "GUID"=w27, "Drop Coords"=w24, "Process Name"=w23) -> (w22:T18)
      n9 = in-place {
        in-place-border: w22 -> [w33]
        n10 = in-place-cluster #1(w18) -> ("Main Config.Feed Module Configs"=w32:T18[])
        n11 = Build Array (concatenate)(w32, w33) -> (w31:T18[])
        n12 = in-place-cluster #1("Main Config.Feed Module Configs"=w31) -> (w17:T2)
      }
      n13 = vi-ref "Feed Module (Main).vi"() -> (w21:refnum<vi>)
      n14 = property class="VI"(reference=w21) -> ("Path"=w20:path)  [unwired: 1 in, 2 out]
      n15 = To Variant(anything=w22) -> (Variant=w25:variant)
      n16 = Bundle By Name(cluster=w26, "Module VI Filepath"=w20, "Module Parameters"=w25, "Process Name"=w23) -> (w28:T66)
    }
    frame "PR" {
      w46 = "PR%d"  # Process Name
      n17 = Format Into String(format string=w46, w36) -> (resulting string=w40:string)  [unwired: 2 in, 1 out]
      n18 = Bundle By Name(cluster=T62 {"GUID"="", "Drop Coords"={"Horizontal"=0, "Vertical"=0}, "Process Name"="", "Queue Name"="", "Settings"={"Cycle Period"=500.0, "PID 2 Parameters"={"Input Device"=enum."Default", "Output Device"=enum."Default", "Setpoint"=0.0, "PID gains"={"proportional gain (Kc)"=1.0, "integral time (Ti, min)"=0.01, "derivative time (Td, min)"=0.0}, "output range"={"output low"=0.0, "output high"=100.0}}, "Manual Entry"=0.0, "Auto?"=TRUE, "4-20mA Input Settings"={"Input Channel "=0}, "4-20mA Out Settings"={"Output DAQ Task"=""}, "Input Channel Tag Name "=""}, "Settings Load Count"=0} ("PRM Config"), "GUID"=w44, "Drop Coords"=w41, "Process Name"=w40) -> (w39:T62)
      n19 = in-place {
        in-place-border: w39 -> [w50]
        n20 = in-place-cluster #2(w35) -> ("Main Config.PR Module Configs"=w49:T62[])
        n21 = Build Array (concatenate)(w49, w50) -> (w48:T62[])
        n22 = in-place-cluster #2("Main Config.PR Module Configs"=w48) -> (w34:T2)
      }
      n23 = vi-ref "4-20mA Module (Main).vi"() -> (w38:refnum<vi>)
      n24 = property class="VI"(reference=w38) -> ("Path"=w37:path)  [unwired: 1 in, 2 out]
      n25 = To Variant(anything=w39) -> (Variant=w42:variant)
      n26 = Bundle By Name(cluster=w43, "Module VI Filepath"=w37, "Module Parameters"=w42, "Process Name"=w40) -> (w45:T66)
    }
    frame "Scale" {
      w63 = "SM%d"  # Process Name
      n27 = Format Into String(format string=w63, w54) -> (resulting string=w57:string)  [unwired: 2 in, 1 out]
      n28 = Bundle By Name(cluster=T40 {"GUID"="", "Drop Coords"={"Horizontal"=0, "Vertical"=0}, "Process Name"="", "Queue Name"="", "Settings"={"Cycle Period"=500.0, "Mettler"={"VISA resource name"="", "Simulated?"=TRUE}, "Scale Type"=""}, "Load Count"=0} ("Scale Module Config"), "GUID"=w61, "Drop Coords"=w58, "Process Name"=w57) -> (w53:T40)
      n29 = in-place {
        in-place-border: w53 -> [w67]
        n30 = in-place-cluster #3(w52) -> ("Main Config.Scale Module Configs"=w66:T40[])
        n31 = Build Array (concatenate)(w66, w67) -> (w65:T40[])
        n32 = in-place-cluster #3("Main Config.Scale Module Configs"=w65) -> (w51:T2)
      }
      n33 = vi-ref "Scale Module (Main).vi"() -> (w56:refnum<vi>)
      n34 = property class="VI"(reference=w56) -> ("Path"=w55:path)  [unwired: 1 in, 2 out]
      n35 = To Variant(anything=w53) -> (Variant=w59:variant)
      n36 = Bundle By Name(cluster=w60, "Module VI Filepath"=w55, "Module Parameters"=w59, "Process Name"=w57) -> (w62:T66)
    }
    frame "Flow" {
      w80 = "FL%d"  # Process Name
      n37 = Format Into String(format string=w80, w71) -> (resulting string=w74:string)  [unwired: 2 in, 1 out]
      n38 = Bundle By Name(cluster=T46 {"GUID"="", "Drop Coords"={"Horizontal"=0, "Vertical"=0}, "Process Name"="", "Queue Name"="", "Settings"={"Cycle Period"=500.0, "Bronkhorst M13"={"VISA resource name"="", "Simulated?"=TRUE}, "Flow Meter Type"="", "Bronkhorst M14"={"VISA resource name"="", "Simulated?"=FALSE}}, "Load Count"=0} ("Scale Module Config"), "GUID"=w78, "Drop Coords"=w75, "Process Name"=w74) -> (w70:T46)
      n39 = in-place {
        in-place-border: w70 -> [w84]
        n40 = in-place-cluster #4(w69) -> ("Main Config.Flow Module Configs"=w83:T46[])
        n41 = Build Array (concatenate)(w83, w84) -> (w82:T46[])
        n42 = in-place-cluster #4("Main Config.Flow Module Configs"=w82) -> (w68:T2)
      }
      n43 = vi-ref "Flow Module.lvlib:Flow Module (Main).vi"() -> (w73:refnum<vi>)
      n44 = property class="VI"(reference=w73) -> ("Path"=w72:path)  [unwired: 1 in, 2 out]
      n45 = To Variant(anything=w70) -> (Variant=w76:variant)
      n46 = Bundle By Name(cluster=w77, "Module VI Filepath"=w72, "Module Parameters"=w76, "Process Name"=w74) -> (w79:T66)
    }
    frame "Pump" {
      w87 = T42 {"GUID"="", "Drop Coords"={"Horizontal"=0, "Vertical"=0}, "Process Name"="", "Queue Name"="", "Settings"={"Cycle Period"=500.0, "Manual Entry"=0.0, "Output Device"=enum."Default", "Ismatech"={"VISA resource name"="", "Simulated?"=TRUE, "Pump Number"=1.0, "Reverse?"=FALSE}, "Masterflex"={"VISA resource name"="", "Simulated?"=TRUE, "Pump Number"=1.0, "Reverse?"=FALSE}, "VICI Settings"={"VISA resource name"="", "Simulated?"=TRUE, "Pump Letter"="", "Reverse?"=FALSE}, "Tacmina Settings"={"Analog DAQ Task"="", "Digital DAQ Task"=""}, "KNF SIMDOS Settings"={"VISA resource name"="", "Simulated?"=TRUE}, "ASIA Pump C"={"ASIA Pump #"=0, "channel"=0, "Simulated"=FALSE}, "FLOM Settings"={"VISA resource name"="", "Simulated?"=TRUE, "Pump Number"=0.0}, "SSI PR/LD Settings"={"VISA resource name"="", "Simulated?"=FALSE}, "SSI P40 Settings"={"VISA resource name"="", "Simulated?"=FALSE}, "Masterflex 75211 Settings"={"Analog DAQ Task"="", "Digital DAQ Task"=""}, "Pump Calibration File"=path "", "Calibration Slope"=0.0, "Calibration Y Intercept"=0.0, "Pump Cal Enum"=0}, "Load Count"=0}  # Pump Module Config
      w98 = "PM%d"  # Process Name
      n47 = Format Into String(format string=w98, w89) -> (resulting string=w92:string)  [unwired: 2 in, 1 out]
      n48 = Bundle By Name(cluster=w87, "GUID"=w96, "Drop Coords"=w93, "Process Name"=w92) -> (w88:T42)
      n49 = in-place {
        in-place-border: w88 -> [w101]
        n50 = in-place-cluster #5(w86) -> ("Main Config.Pump Module Configs"=w100:T42[])
        n51 = Build Array (concatenate)(w100, w101) -> (w99:T42[])
        n52 = in-place-cluster #5("Main Config.Pump Module Configs"=w99) -> (w85:T2)
      }
      n53 = vi-ref "Pump Module (Main).vi"() -> (w91:refnum<vi>)
      n54 = property class="VI"(reference=w91) -> ("Path"=w90:path)  [unwired: 1 in, 2 out]
      n55 = To Variant(anything=w88) -> (Variant=w94:variant)
      n56 = Bundle By Name(cluster=w95, "Module VI Filepath"=w90, "Module Parameters"=w94, "Process Name"=w92) -> (w97:T66)
    }
    frame "DO" {
      w104 = T57 {"GUID"="", "Drop Coords"={"Horizontal"=0, "Vertical"=0}, "Process Name"="", "Queue Name"="", "Settings"={"Valve Settings"={"D-O Settings"={"DAQmx Task Name"="", "Output Channel"=0, "Output Channel Names"=[]}, "VICI Electronic Actuator"={"VISA resource name"="", "Mode"=enum."Two Positions With Stops", "Simulated"=FALSE}}, "Valve Type"=enum."Default", "Time On (Sec)"=0.0, "Time Off (Sec)"=0.0, "Run?"=FALSE}, "Load Count"=0}  # D-O Module Config
      w115 = "DO%d"  # Process Name
      # "DO Module (Main).vit"
      n57 = Format Into String(format string=w115, w106) -> (resulting string=w109:string)  [unwired: 2 in, 1 out]
      n58 = Bundle By Name(cluster=w104, "GUID"=w113, "Drop Coords"=w110, "Process Name"=w109) -> (w105:T57)
      n59 = in-place {
        in-place-border: w105 -> [w118]
        n60 = in-place-cluster #6(w103) -> ("Main Config.DO Module Configs"=w116:T57[])
        n61 = Build Array (concatenate)(w116, w118) -> (w117:T57[])
        n62 = in-place-cluster #6("Main Config.DO Module Configs"=w117) -> (w102:T2)
      }
      n63 = vi-ref "D-O Module.lvlib:D-O Module (Main).vi"() -> (w108:refnum<vi>)
      n64 = property class="VI"(reference=w108) -> ("Path"=w107:path)  [unwired: 1 in, 2 out]
      n65 = To Variant(anything=w105) -> (Variant=w111:variant)
      n66 = Bundle By Name(cluster=w112, "Module VI Filepath"=w107, "Module Parameters"=w111, "Process Name"=w109) -> (w114:T66)
    }
    frame "TCU" {
      w121 = T48 {"GUID"="", "Drop Coords"={"Horizontal"=0, "Vertical"=0}, "Process Name"="", "Queue Name"="", "Settings"={"Cycle Period"=500.0, "Setpoint Entry"=0.0, "Output Device"=enum."Default", "Huber Ministat 230 Settings"={"VISA resource name"="", "Simulated?"=FALSE}, "Lauda Settings"={"VISA resource name"="", "Simulated?"=FALSE, "Pump Power"=2}, "Julabo FP-50 Settings"={"VISA resource name"="", "Simulated?"=FALSE, "Pump Power"=2}, "Internal Control?"=FALSE, "Huber Unistat 410 Settings"={"VISA resource name"="", "Address"=0, "Simulated?"=FALSE}}, "Load Count"=0, "Power Level Changed"=FALSE}  # TCU Module Config
      w132 = "TC%d"  # Process Name
      # "Pump Module (Main).vit"
      n67 = Format Into String(format string=w132, w123) -> (resulting string=w126:string)  [unwired: 2 in, 1 out]
      n68 = Bundle By Name(cluster=w121, "GUID"=w130, "Drop Coords"=w127, "Process Name"=w126) -> (w122:T48)
      n69 = in-place {
        in-place-border: w122 -> [w135]
        n70 = in-place-cluster #7(w120) -> ("Main Config.TCU Module Configs"=w134:T48[])
        n71 = Build Array (concatenate)(w134, w135) -> (w133:T48[])
        n72 = in-place-cluster #7("Main Config.TCU Module Configs"=w133) -> (w119:T2)
      }
      n73 = vi-ref "TCU Module.lvlib:TCU Module (Main).vi"() -> (w125:refnum<vi>)
      n74 = property class="VI"(reference=w125) -> ("Path"=w124:path)  [unwired: 1 in, 2 out]
      n75 = To Variant(anything=w122) -> (Variant=w128:variant)
      n76 = Bundle By Name(cluster=w129, "Module VI Filepath"=w124, "Module Parameters"=w128, "Process Name"=w126) -> (w131:T66)
    }
    frame "TT" {
      w150 = "TT%d"  # Prefix
      # "TT (Main).vit"
      n77 = Format Into String(format string=w150, w139) -> (resulting string=w144:string)  [unwired: 2 in, 1 out]
      n78 = call "Default Numeric Alarms (TT).vi"() -> ("Default Numeric Alarms"=w138:T36[])  [unwired: 11 in]
      n79 = Bundle By Name(cluster=T35 {"GUID"="", "Drop Coords"={"Horizontal"=0, "Vertical"=0}, "Input Channel Tag Name "="", "Process Name"="", "Queue Name"="", "Input Channel Numeric Alarm Settings"=[]} ("TT Module Config"), "GUID"=w148, "Drop Coords"=w145, "Process Name"=w144, "Input Channel Numeric Alarm Settings"=w138) -> (w142:T35)
      n80 = in-place {
        in-place-border: w142 -> [w153]
        n81 = in-place-cluster #8(w136) -> ("Main Config.TT Module Configs"=w152:T35[])
        n82 = Build Array (concatenate)(w152, w153) -> (w151:T35[])
        n83 = in-place-cluster #8("Main Config.TT Module Configs"=w151) -> (w137:T2)
      }
      n84 = vi-ref "TT (Main).vi"() -> (w141:refnum<vi>)
      n85 = property class="VI"(reference=w141) -> ("Path"=w140:path)  [unwired: 1 in, 2 out]
      n86 = To Variant(anything=w142) -> (Variant=w146:variant)
      n87 = Bundle By Name(cluster=w147, "Module VI Filepath"=w140, "Module Parameters"=w146, "Process Name"=w144) -> (w149:T66)
    }
    frame "U3" {
      w168 = "U3%d"  # Prefix
      # "U3 (Main).vit"
      n88 = Format Into String(format string=w168, w157) -> (resulting string=w162:string)  [unwired: 2 in, 1 out]
      n89 = call "Default Numeric Alarms (TT).vi"() -> ("Default Numeric Alarms"=w156:T36[])  [unwired: 11 in]
      n90 = Bundle By Name(cluster=T44 {"GUID"="", "Drop Coords"={"Horizontal"=0, "Vertical"=0}, "AI Channel Number"=enum."Default", "Process Name"="", "Queue Name"="", "Input Channel Numeric Alarm Settings"=[]} ("TT Module Config"), "GUID"=w166, "Drop Coords"=w163, "Process Name"=w162, "Input Channel Numeric Alarm Settings"=w156) -> (w160:T44)
      n91 = in-place {
        in-place-border: w160 -> [w171]
        n92 = in-place-cluster #9(w155) -> ("Main Config.U3 Module Configs"=w170:T44[])
        n93 = Build Array (concatenate)(w170, w171) -> (w169:T44[])
        n94 = in-place-cluster #9("Main Config.U3 Module Configs"=w169) -> (w154:T2)
      }
      n95 = vi-ref "U3 Module.lvlib:U3 (Main).vit"() -> (w159:refnum<vi>)
      n96 = property class="VI"(reference=w159) -> ("Path"=w158:path)  [unwired: 1 in, 2 out]
      n97 = To Variant(anything=w160) -> (Variant=w164:variant)
      n98 = Bundle By Name(cluster=w165, "Module VI Filepath"=w158, "Module Parameters"=w164, "Process Name"=w162) -> (w167:T66)
    }
    frame "PT" {
      w186 = "PT%d"  # Process Name
      n99 = Format Into String(format string=w186, w175) -> (resulting string=w180:string)  [unwired: 2 in, 1 out]
      n100 = call "Default Numeric Alarms (TT).vi"() -> ("Default Numeric Alarms"=w174:T36[])  [unwired: 11 in]
      n101 = Bundle By Name(cluster=T39 {"GUID"="", "Drop Coords"={"Horizontal"=0, "Vertical"=0}, "Input Channel Tag Name "="", "Process Name"="", "Queue Name"="", "Input Channel Numeric Alarm Settings"=[]} ("TT Module Config"), "GUID"=w184, "Drop Coords"=w181, "Process Name"=w180, "Input Channel Numeric Alarm Settings"=w174) -> (w178:T39)
      n102 = in-place {
        in-place-border: w178 -> [w189]
        n103 = in-place-cluster #10(w173) -> ("Main Config.PT Module Configs"=w188:T39[])
        n104 = Build Array (concatenate)(w188, w189) -> (w187:T39[])
        n105 = in-place-cluster #10("Main Config.PT Module Configs"=w187) -> (w172:T2)
      }
      n106 = vi-ref "PT (Main).vi"() -> (w177:refnum<vi>)
      n107 = property class="VI"(reference=w177) -> ("Path"=w176:path)  [unwired: 1 in, 2 out]
      n108 = To Variant(anything=w178) -> (Variant=w182:variant)
      n109 = Bundle By Name(cluster=w183, "Module VI Filepath"=w176, "Module Parameters"=w182, "Process Name"=w180) -> (w185:T66)
    }
    frame "OPC" {
      n110 = in-place {
        in-place-border: w196 -> [w209]
        in-place-border: w195 -> [w208]
        in-place-border: w194 -> [w206]
        in-place-border: w193 -> [w202]
        in-place-border: [w199] -> w192
        w210 = "OP%d"  # Process Name
        n111 = in-place-cluster #11(w191) -> ("Main Config.OPC Module Configs"=w198:T9[])
        n112 = Format Into String(format string=w210, w202) -> (resulting string=w205:string)  [unwired: 2 in, 1 out]
        n113 = Bundle By Name(cluster=T9 {"State"=enum."Idle", "GUID"="", "Drop Coords"={"Horizontal"=0, "Vertical"=0}, "Configuration"={"Cycle Period"=500.0, "server endpoint URL"="", "security policy"={"message mode"=enum."None", "security"=enum."Basic256"}, "Trust Any Server"=TRUE}, "First Iteration"=FALSE, "Data"=[], "Process Name"="", "Load Count"=0, "Log Started"=FALSE, "subscription ID out"=0, "OPC UA client refnum out"="", "Event Registration Refnum"=refnum, "Start Time"=timestamp(0 s since 1904-01-01), "Current Time"=timestamp(0 s since 1904-01-01)} ("OPC Module Config"), "GUID"=w209, "Drop Coords"=w206, "Process Name"=w205) -> (w204:T9)
        n114 = vi-ref "OPC Main.vi"() -> (w201:refnum<vi>)
        n115 = property class="VI"(reference=w201) -> ("Path"=w203:path)  [unwired: 1 in, 2 out]
        n116 = To Variant(anything=w204) -> (Variant=w207:variant)
        n117 = Build Array (concatenate)(w198, w204) -> (w197:T9[])
        n118 = in-place-cluster #11("Main Config.OPC Module Configs"=w197) -> (w190:T2)
        n119 = Bundle By Name(cluster=w208, "Module VI Filepath"=w203, "Module Parameters"=w207, "Process Name"=w205) -> (w199:T66)
      }
    }
    frame Default {
      # "This case should not execute."
    }
  }
  "Drop Parameters" <- w16
  "State out" <- w2
